vi "频率测量.vi"(11 "采样数":i32=4000) -> ()   [LabVIEW 2010]
doc: "Creates, edits, and runs tasks using NI-DAQmx. Refer to the DAQ Quick Start Guide for information on devices supported by NI-DAQmx.\n\nWhen you place this Express VI on the block diagram, the DAQ Assistant launches to create a new task. After you create a task, you can double-click the DAQ Assistant Express VI in order to edit that task. For continuous measurement or generation, place a loop around the DAQ Assistant Express VI. \n\nFor continuous single-point input or output, the DAQ Assistant Express VI might not provide satisfactory performance. Refer to examples\\DAQmx\\Analog In\\Measure Voltage.llb\\Cont Acq&Graph Voltage-Single Point Optimization.vi for techniques to create higher-performance, single-point I/O applications."
uses:
  <vilib>/DAQmx/read.llb/DAQmx Read.vi
  <vilib>/DAQmx/read.llb/DAQmx Read (Analog 1D DBL 1Chan NSamp).vi
  <vilib>/DAQmx/create/channels.llb/DAQmx Create Channel (AI-Voltage-Basic).vi
  <vilib>/DAQmx/configure/timing.llb/DAQmx Timing (Sample Clock).vi
  <vilib>/Analysis/4window.llb/Hanning Window (DBL).vi
  <vilib>/daqmx/miscellaneous.llb/DAQmx Fill In Error Info.vi
  <vilib>/Analysis/NI_AALPro.lvlib
panel:
  out "频谱":dbl[](graph)
  in  "停止":bool
  in  "rate":dbl=4000.0
  out "波形图":dbl[](graph)
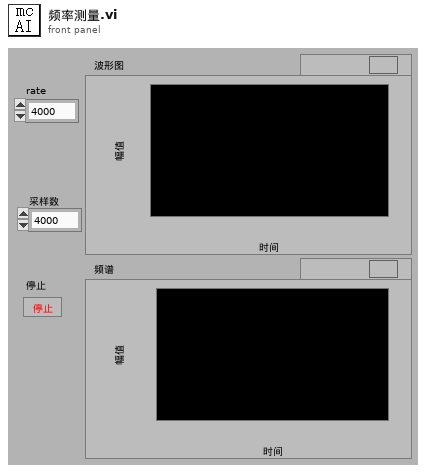
[diagram p1: front panel]
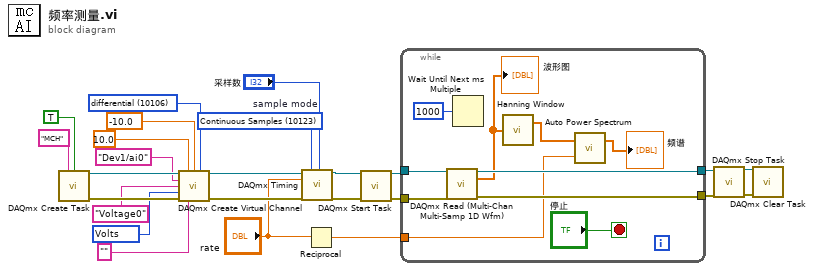
[diagram p0: block diagram]
diagram:
  w7 = 10348 items=["Volts"=10348, "From Custom Scale"=10065] ("units")
  w12 = 10106 items=["default"=-1, "differential"=10106, "RSE"=10083, "NRSE"=10078] ("input terminal configuration")
  w21 = 10123 items=["Finite Samples"=10178, "Continuous Samples"=10123, "Hardware Timed Single Point"=12522]  # sample mode
  n1 = call <vilib>:"DAQmx Create Task.vi"("new task name"="MCH", "auto cleanup"=TRUE) -> ("task out"=w25:refnum<k21>, "error out"=w24:errorcluster)  [unwired: 12 in]
  n2 = call-poly <vilib>:"DAQmx Create Virtual Channel.vi"("task in"=w25, "maximum value"=10.0, "minimum value"=-10.0, "input terminal configuration"=w12, "physical channels"="Dev1/ai0" ("physical channel"), "name to assign"="Voltage0" ("channel name"), "units"=w7, "error in"=w24, "custom scale name"="") -> ("task out"=w23:refnum<k21>, "error out"=w22:errorcluster)  [unwired: 5 in]
  n3 = call-poly <vilib>:"DAQmx Timing.vi"("task/channels in"=w23, "sample mode"=w21, "samples per channel"="采样数", "rate"="rate", "error in"=w22) -> ("task out"=w14:refnum<k21>, "error out"=w13:errorcluster)  [unwired: 9 in]
  n4 = Reciprocal(x="rate") -> (1/x=w1:dbl)
  n5 = call <vilib>:"DAQmx Start Task.vi"("task/channels in"=w14, "error in"=w13) -> ("task out"=w5:refnum<k21>, "error out"=w4:errorcluster)  [unwired: 12 in]
  n6 = while {
    tunnel: [w35] -> w20
    tunnel: [w34] -> w19
    tunnel: w5 -> [w33]
    tunnel: w4 -> [w32]
    tunnel: w1 -> [w29]
    stop <- "停止" stop-if-true
    n7 = call-poly "DAQmx Read (Multi-Chan Multi-Samp 1D Wfm).vi"("task/channels in"=w33, "error in"=w32) -> ("task out"=w34:refnum<k21>, "data"=w27:dbl[], "error out"=w35:errorcluster)  [unwired: 11 in]
    "波形图" <- w27
    n8 = Wait Until Next ms Multiple(millisecond multiple=u32 1000 ("毫秒倍数")) -> ()  [unwired: 1 out]
    n9 = call-poly <vilib>:"Hanning Window.vi"("X"=w27) -> ("Windowed X"=w26:dbl[])  [unwired: 1 out]
    n10 = call <vilib>:"Auto Power Spectrum.vi"("dt"=w29, "Signal (V)"=w26) -> ("Power Spectrum (V^2 rms)"=→"频谱":dbl[])  [unwired: 1 out]
  }
  n11 = call <vilib>:"DAQmx Stop Task.vi"("task/channels in"=w19, "error in"=w20) -> ("task out"=w18:refnum<k21>, "error out"=w17:errorcluster)  [unwired: 12 in]
  n12 = call <vilib>:"DAQmx Clear Task.vi"("task in"=w18, "error in"=w17) -> ()  [unwired: 13 in, 1 out]
